vi "Settings Dialog.vi"(8 "error in (no error)":errorcluster, 11 "Settings in":T1={"Logging Configuration"={"Log File Base Path"=path "", "Samples to Save"=0, "Acquisition Sample Rate"=0.0, "SamplesPerChannel"=0, "FFT - Block Size"=0, "FFT - NumberOfAverages"=0, "Trigger - Time"=0, "Trigger - Threshold"=0.0, "Trigger - Channel"=0, "Enable Start Output Trigger"=FALSE, "Enable Time Trigger"=FALSE, "Enable Threshold Trigger"=FALSE, "HasBeenTriggeredAlready"=FALSE, "Always Log"=FALSE, "Enable Filter"=FALSE, "FilesRefs"={"TimeDomainTDMSRef"=refnum, "FrequencyDomainTDMSRef"=refnum, "TimeDomainTXTRef"=refnum, "FrequencyDomainTXTRef "=refnum}, "OutputFileFormat"=enum."TXT", "ActualBlockSize"=0, "Start Time"=timestamp(0 s since 1904-01-01)}, "Hardware Configuration"={"Accel-ai0"=FALSE, "Maximum Input"=0.0, "Minimum Input"=0.0, "HW Sample Rate"=0.0, "SW Sample Rate"=0.0, "Number of Samples"=0, "Accel-ai1"=FALSE, "DAQmx Task"="", "Low Pass Filter"={"Upper Cutoff"=350.0, "Lower Cutoff"=350.0, "Order"=350}}, "Output Hardware Configuration"={"Task ID"=0, "Volume"=0.0, "Sample Rate"=0.0, "Duration"=0, "Data"={"SignalType"=enum."SineWave", "Amplitude"=0.0, "WhiteNoiseSettings"={"Generate New Data"=FALSE, "Save"=FALSE, "Filter"=TRUE, "Gain"=0.0}, "SineWaveSttings"={"Frequency"=0.0}}, "Generated Data"={"t0"=timestamp(0 s since 1904-01-01), "dt"=1.0, "Y"=[]}}} {"Output Hardware Configuration"."task ID out" format="%.0x"; "Hardware Configuration"."Low Pass Filter"."Order" min=0 max=10 step=1}) -> (0 "error out":errorcluster, 1 "Cancelled?":bool=TRUE, 2 "UI Refresh Needed?":bool, 3 "Settings Out":T1={"Logging Configuration"={"Log File Base Path"=path "", "Samples to Save"=0, "Acquisition Sample Rate"=0.0, "SamplesPerChannel"=0, "FFT - Block Size"=0, "FFT - NumberOfAverages"=0, "Trigger - Time"=0, "Trigger - Threshold"=0.0, "Trigger - Channel"=0, "Enable Start Output Trigger"=FALSE, "Enable Time Trigger"=FALSE, "Enable Threshold Trigger"=FALSE, "HasBeenTriggeredAlready"=FALSE, "Always Log"=FALSE, "Enable Filter"=FALSE, "FilesRefs"={"TimeDomainTDMSRef"=refnum, "FrequencyDomainTDMSRef"=refnum, "TimeDomainTXTRef"=refnum, "FrequencyDomainTXTRef "=refnum}, "OutputFileFormat"=enum."TXT", "ActualBlockSize"=0, "Start Time"=timestamp(0 s since 1904-01-01)}, "Hardware Configuration"={"Accel-ai0"=FALSE, "Maximum Input"=0.0, "Minimum Input"=0.0, "HW Sample Rate"=0.0, "SW Sample Rate"=0.0, "Number of Samples"=0, "Accel-ai1"=FALSE, "DAQmx Task"="", "Low Pass Filter"={"Upper Cutoff"=350.0, "Lower Cutoff"=350.0, "Order"=350}}, "Output Hardware Configuration"={"Task ID"=0, "Volume"=0.0, "Sample Rate"=0.0, "Duration"=0, "Data"={"SignalType"=enum."SineWave", "Amplitude"=0.0, "WhiteNoiseSettings"={"Generate New Data"=FALSE, "Save"=FALSE, "Filter"=TRUE, "Gain"=0.0}, "SineWaveSttings"={"Frequency"=0.0}}, "Generated Data"={"t0"=timestamp(0 s since 1904-01-01), "dt"=1.0, "Y"=[]}}} {"Output Hardware Configuration"."task ID out" format="%.0x"; "Hardware Configuration"."Low Pass Filter"."Order" min=0 max=10 step=1})   [LabVIEW 2022 SP3, in "Settings.lvlib"]
doc: "Dialog for selecting user specified settings."
uses:
  Settings.lvlib
  Settings.ctl
  Logging/Logging Configuration.ctl
  support/TDMS-Refs.ctl
  FiniteMeasurement-DAQmx/controls/Hardware Configuration.ctl
  AcquisitionFilter.ctl
  Output/Output Hardware Configuration.ctl
  <vilib>/sound2/lvsound2.llb/Sound Output Task ID.ctl
  Output/Data.ctl
  Output/WhiteNoiseSettings.ctl
  Output/SineWaveSettings.ctl
  <vilib>/Utility/xml.llb/Write to XML File(string).vi
  <resource>/objmgr/daqmx.rc
  Logging/Logging.lvlib
  Acquisition/Acquisition.lvlib
panel:
  out "Frequency Delta(Hz)":dbl
  in  "Logging Configuration.Enable Filter":bool
  in  "Lower Cutoff":dbl
  in  "Order":i32
  in  "Number of FFT Averages":i32=5
  in  "Block Size":u32=100 min=100 max=10240 step=10
  in  "Accelerometer AI-1":bool
  in  "Accelerometer AI-0":bool=TRUE
  in  "Log when triggered":bool
  in  "Trigger Channel":u32
  in  "Timeout (s)":u32=206000 min=1
  in  "Trigger Threshold (V)":dbl=2.0
  in  "Trigger Time (s)":u32=1
  in  "Enable Threshold Trigger (m/s²):":bool
  in  "Enable Time Trigger (s):":bool
  in  "Always Log":bool
  in  "HW Sample Rate":i32=20000 min=1000 max=20000
  in  "SW Sample Rate":dbl=220.0
  in  "Max/Min Input":dbl=5.0
  in  "Log Base Path":path=path "C:/Users/LAV-UFSC-2023/Documents/LAV-TCC/Dados-Experimentos/Dados-Bancada-LABVIEW/teste.txt"
  in  "Cancel Button":bool
  in  "OK Button":bool
  # "Acquisition"
  # "Non visible portion of dialog (needed for connector pane)."
  # "LowPassFilter"
  # "Trigger"
  # "Logging"
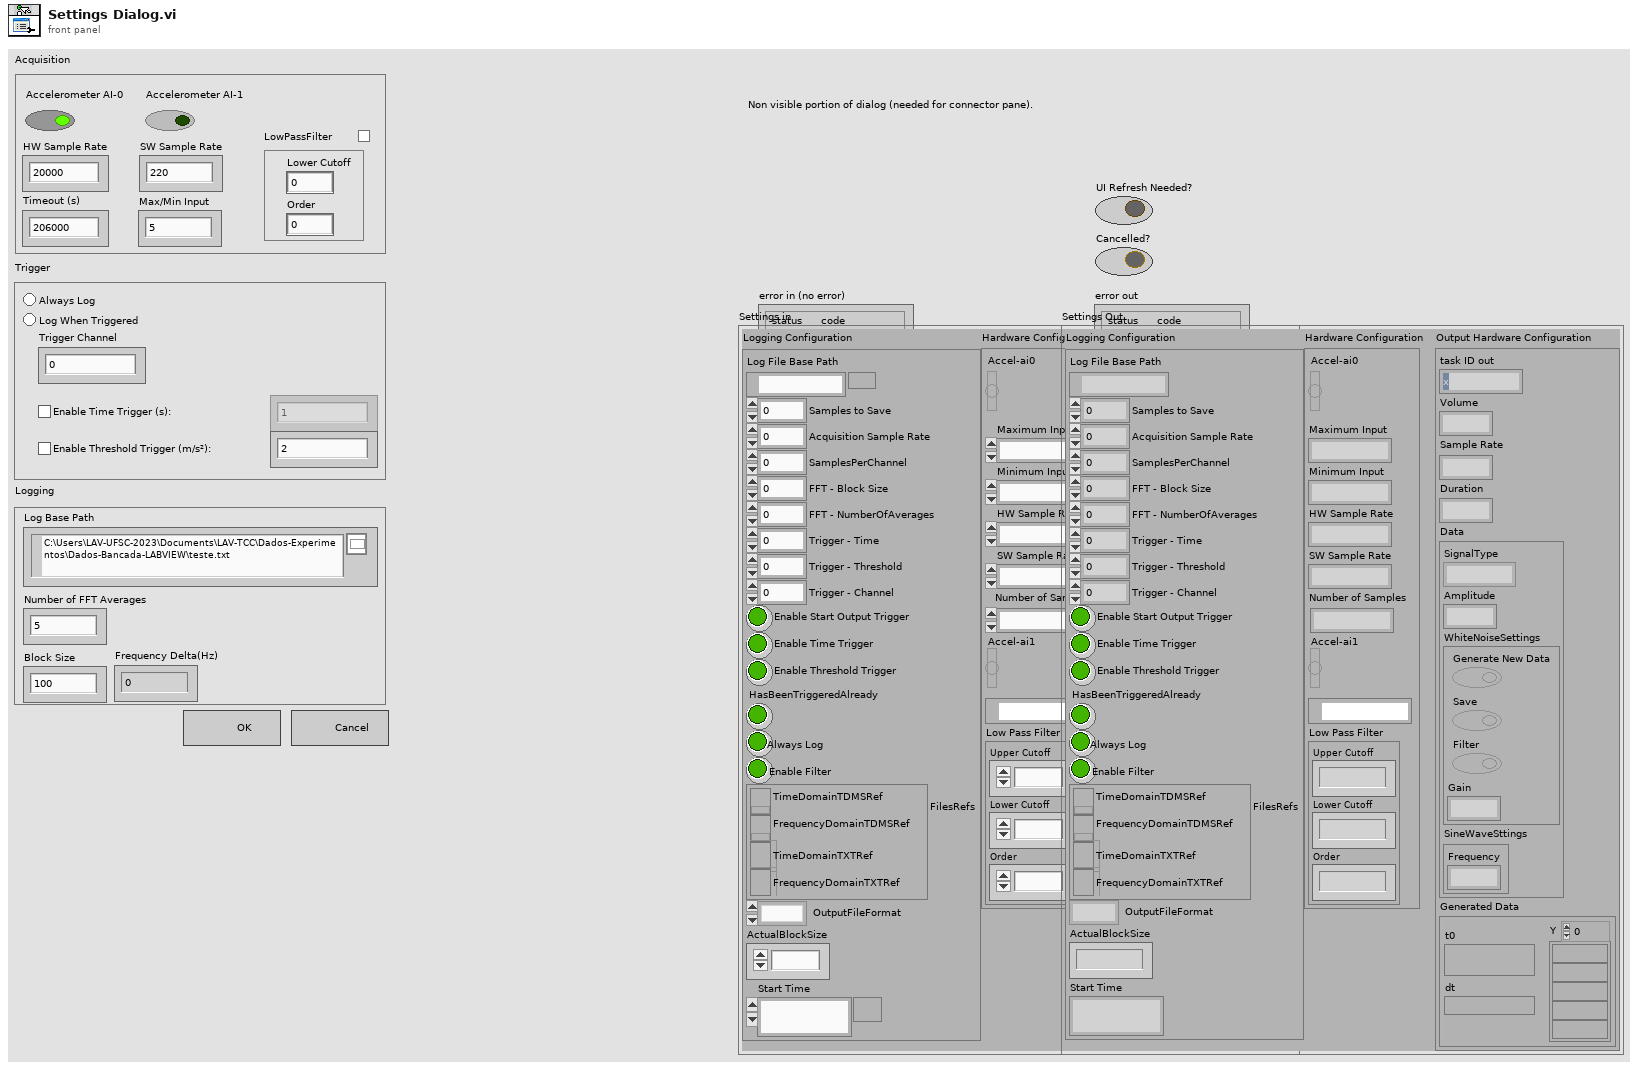
[diagram p1: front panel]
types:
  T1 = typedef "Settings.lvlib/Settings.ctl" = cluster{"Logging Configuration":T2, "Hardware Configuration":T4, "Output Hardware Configuration":T6}
  T2 = typedef "Logging.lvlib/Logging Configuration.ctl" = cluster{"Log File Base Path":path, "Samples to Save":u32, "Acquisition Sample Rate":dbl, "SamplesPerChannel":u32, "FFT - Block Size":u32, "FFT - NumberOfAverages":i32, "Trigger - Time":i32, "Trigger - Threshold":dbl, "Trigger - Channel":i32, "Enable Start Output Trigger":bool, "Enable Time Trigger":bool, "Enable Threshold Trigger":bool, "HasBeenTriggeredAlready":bool, "Always Log":bool, "Enable Filter":bool, "FilesRefs":T3, "OutputFileFormat":enum16{"TXT", "TDMS"}, "ActualBlockSize":i32, "Start Time":timestamp}
  T3 = typedef "TDMS-Refs.ctl" = cluster{"TimeDomainTDMSRef":refnum<k34>, "FrequencyDomainTDMSRef":refnum<k34>, "TimeDomainTXTRef":refnum<file>, "FrequencyDomainTXTRef ":refnum<file>}
  T4 = typedef "Acquisition.lvlib/Hardware Configuration.ctl" = cluster{"Accel-ai0":bool, "Maximum Input":dbl, "Minimum Input":dbl, "HW Sample Rate":dbl, "SW Sample Rate":dbl, "Number of Samples":i32, "Accel-ai1":bool, "DAQmx Task":refnum<k21>, "Low Pass Filter":T5}
  T5 = typedef "Acquisition.lvlib/AcquisitionFilter.ctl" = cluster{"Upper Cutoff":dbl, "Lower Cutoff":dbl, "Order":i32}
  T6 = typedef "Output Hardware Configuration.ctl" = cluster{"Task ID":T7, "Volume":dbl, "Sample Rate":dbl, "Duration":i32, "Data":T8, "Generated Data":waveform(dbl)}
  T7 = typedef "Sound Output Task ID.ctl" = u32
  T8 = typedef "Data.ctl" = cluster{"SignalType":enum16{"WhiteNoise", "SineWave"}, "Amplitude":dbl, "WhiteNoiseSettings":T9, "SineWaveSttings":T10}
  T9 = typedef "WhiteNoiseSettings.ctl" = cluster{"Generate New Data":bool, "Save":bool, "Filter":bool, "Gain":dbl}
  T10 = typedef "SineWaveSettings.ctl" = cluster{"Frequency":dbl}
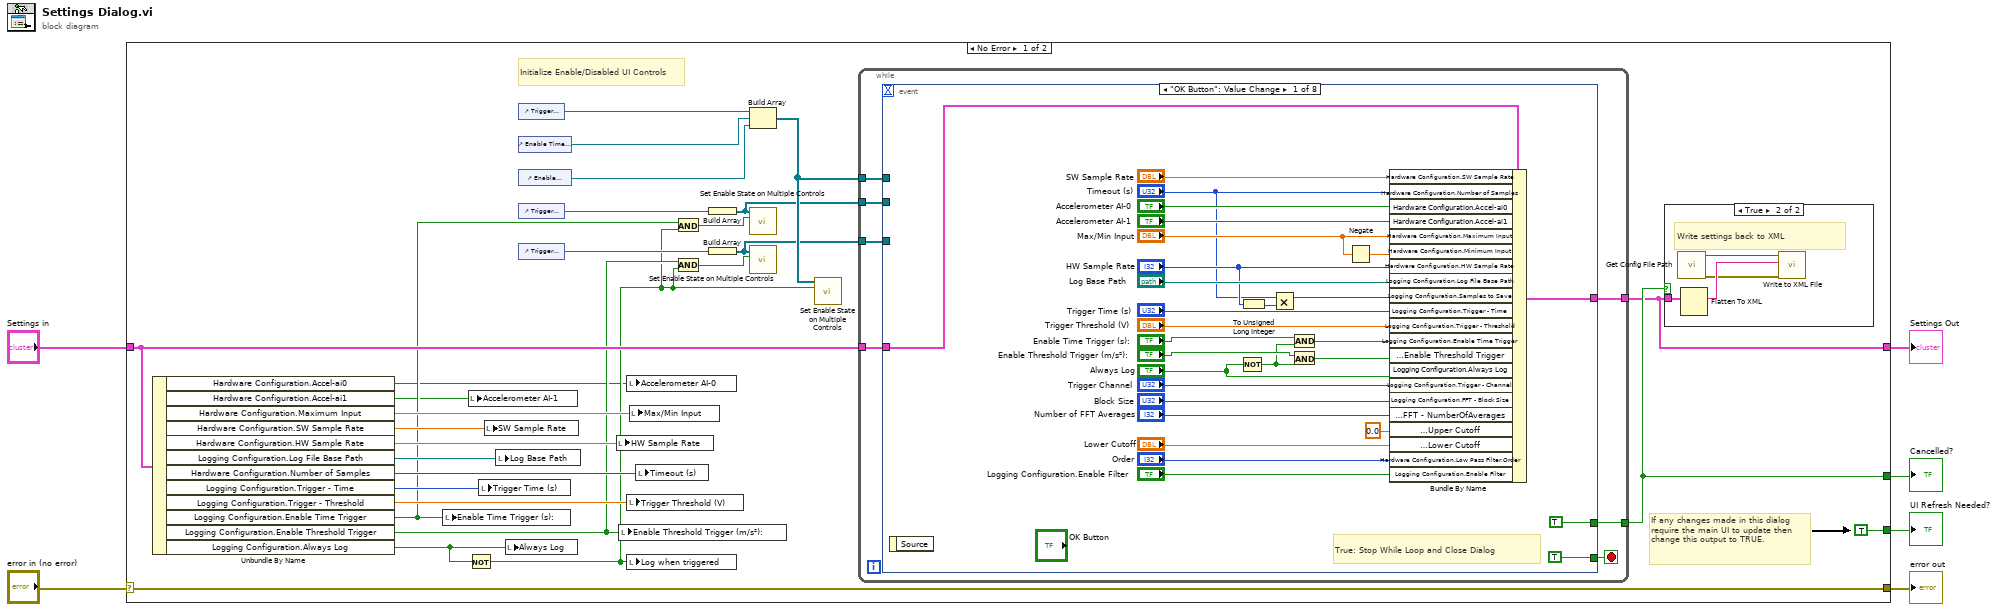
[diagram p0: block diagram]
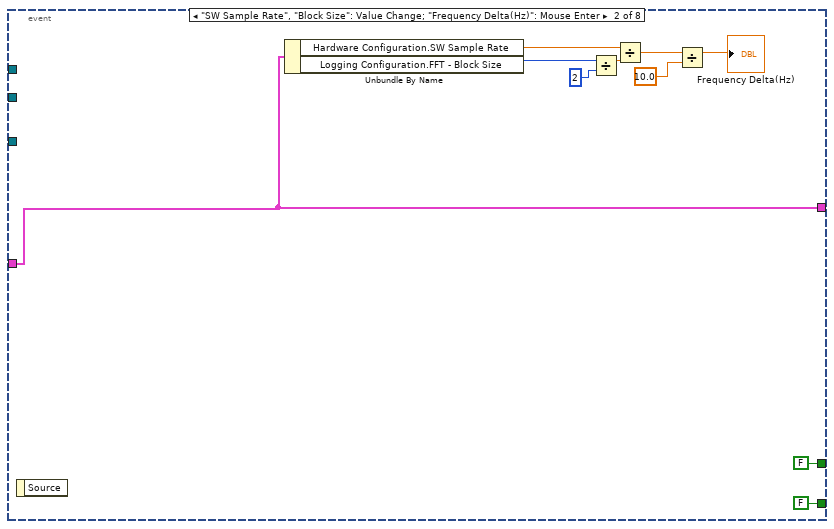
[diagram p2: hidden frame]
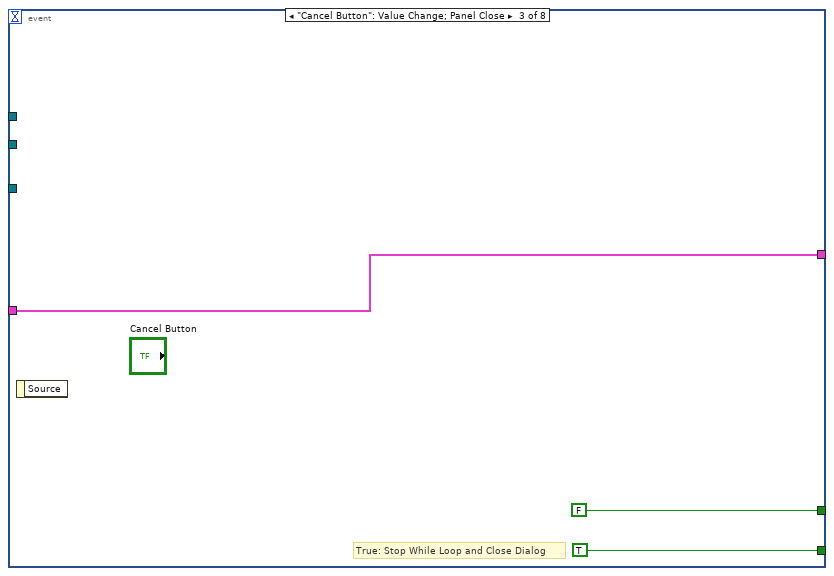
[diagram p3: hidden frame]
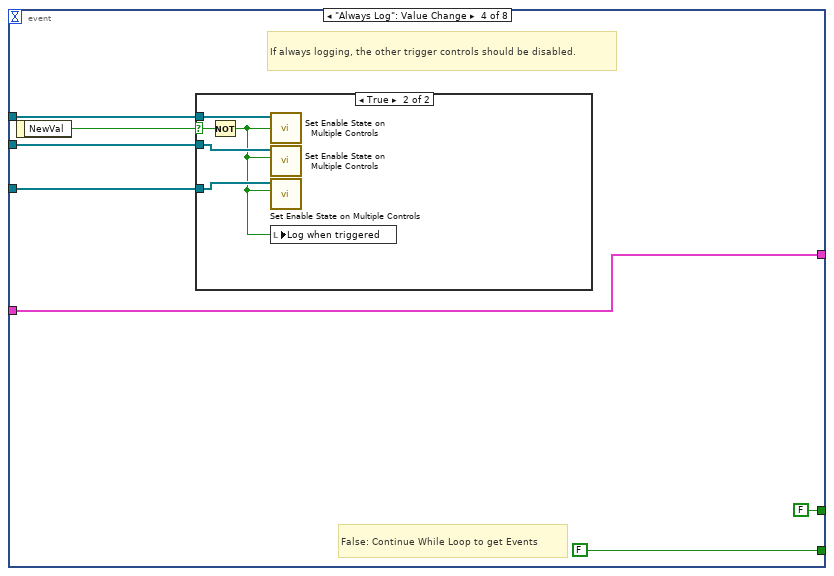
[diagram p4: hidden frame]
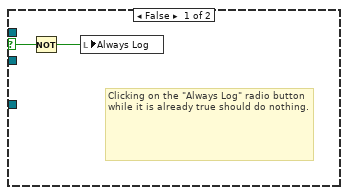
[diagram p5: hidden frame]
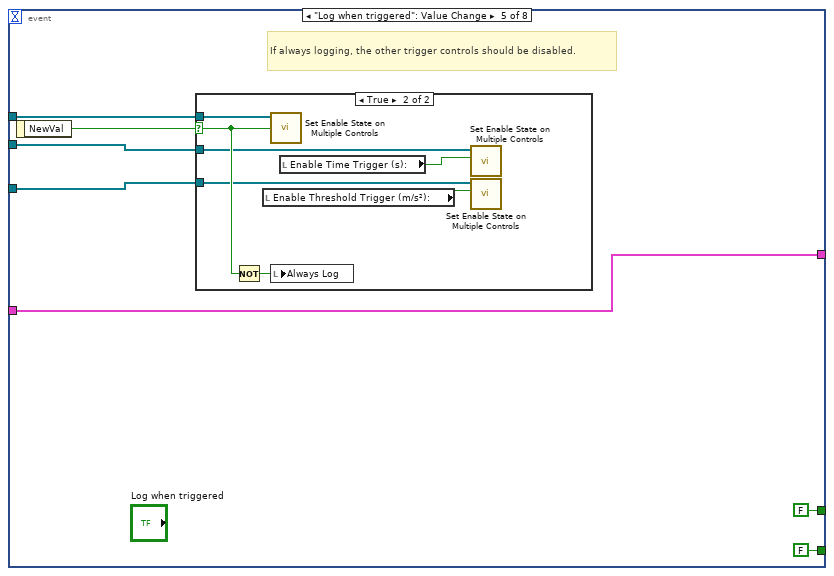
[diagram p6: hidden frame]
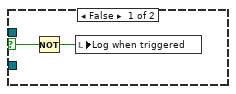
[diagram p7: hidden frame]
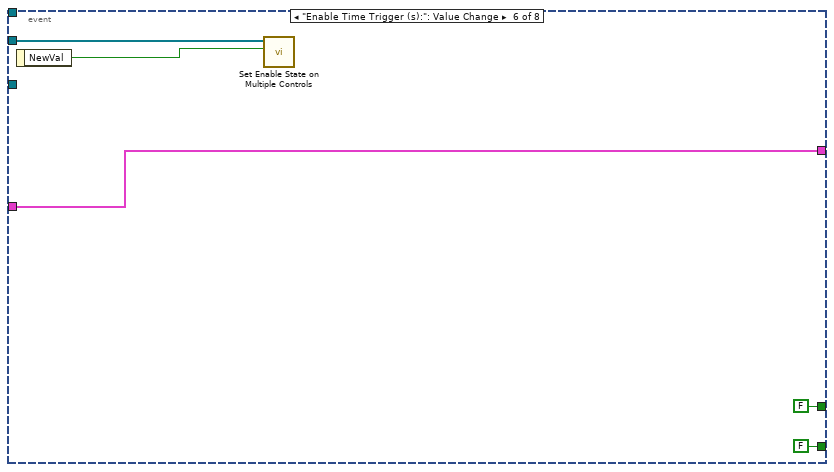
[diagram p8: hidden frame]
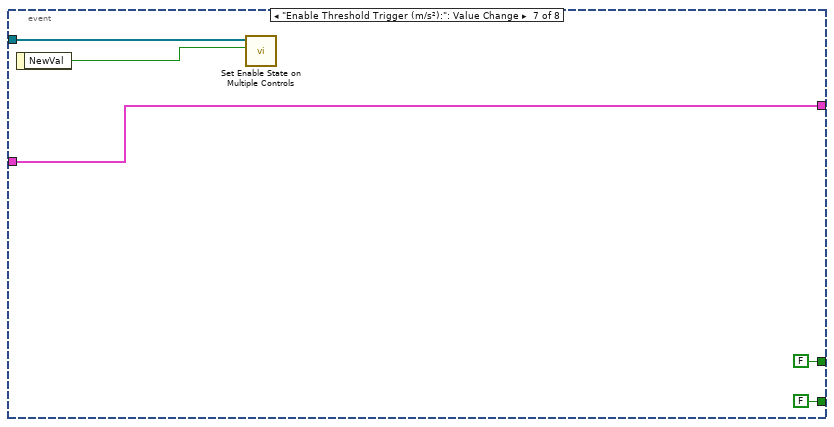
[diagram p9: hidden frame]
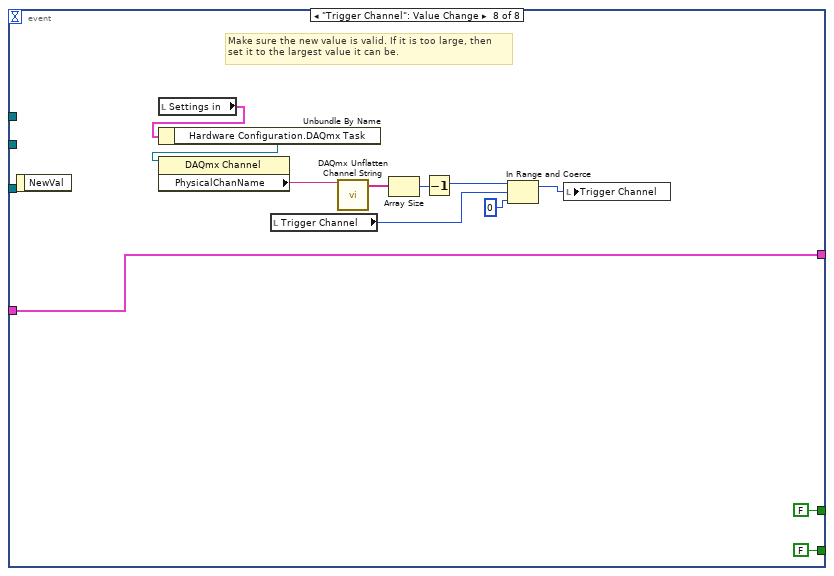
[diagram p10: hidden frame]
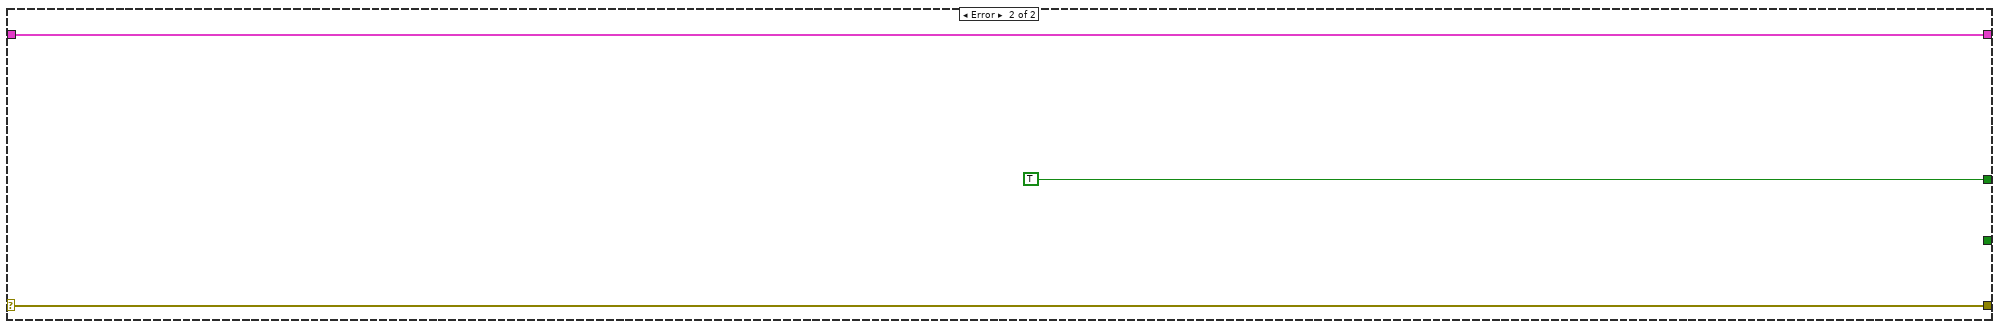
[diagram p12: hidden frame]
diagram:
  n1 = case shown="No Error" "error in (no error)" {
    selector: "error in (no error)" -> [w34 w142]
    tunnel: [w34 w142] -> w6
    tunnel: "Settings in" -> [w21 w141]
    tunnel: [w31 w141] -> w5
    tunnel: [TRUE ("UI Refresh Needed?") _] -> w4
    tunnel: [w32 TRUE ("UI Refresh Needed?")] -> w3
    frame No Error {
      # "Initialize Enable/Disabled UI Controls"
      # "If any changes made in this dialog require the main UI to update then change this output to TRUE."
      n2 = Unbundle By Name(w21) -> ("Hardware Configuration.Accel-ai0"=w7:bool, "Hardware Configuration.Accel-ai1"=w8:bool, "Hardware Configuration.Maximum Input"=w28:dbl, "Hardware Configuration.SW Sample Rate"=w29:dbl, "Hardware Configuration.HW Sample Rate"=w30:dbl, "Logging Configuration.Log File Base Path"=w27:path, "Hardware Configuration.Number of Samples"=w26:i32, "Logging Configuration.Trigger - Time"=w25:i32, "Logging Configuration.Trigger - Threshold"=w24:dbl, "Logging Configuration.Enable Time Trigger"=w13:bool, "Logging Configuration.Enable Threshold Trigger"=w12:bool, "Logging Configuration.Always Log"=w23:bool)
      n3 = local write "Enable Time Trigger (s):"(w13) -> ()
      n4 = Not(x=w23) -> (.not. x?=w9:bool)
      n5 = local write "Accelerometer AI-1"(w8) -> ()
      n6 = local write "Trigger Time (s)"(w25) -> ()
      n7 = local write "SW Sample Rate"(w29) -> ()
      n8 = local write "Log Base Path"(w27) -> ()
      n9 = local write "Always Log"(w23) -> ()
      n10 = control-ref of="Trigger Channel"() -> (w20:refnum<vi>)
      n11 = control-ref of="Enable Time Trigger (s):"() -> (w19:refnum<vi>)
      n12 = control-ref of="Enable Threshold Trigger (m/s²):"() -> (w18:refnum<vi>)
      n13 = control-ref of="Trigger Time (s)"() -> (w17:refnum<vi>)
      n14 = control-ref of="Trigger Threshold (V)"() -> (w16:refnum<vi>)
      n15 = local write "HW Sample Rate"(w30) -> ()
      n16 = local write "Enable Threshold Trigger (m/s²):"(w12) -> ()
      n17 = local write "Accelerometer AI-0"(w7) -> ()
      n18 = local write "Trigger Threshold (V)"(w24) -> ()
      n19 = local write "Log when triggered"(w9) -> ()
      n20 = local write "Max/Min Input"(w28) -> ()
      n21 = local write "Timeout (s)"(w26) -> ()
      n22 = And(x=w13, y=w9) -> (x .and. y?=w15:bool)
      n23 = And(x=w12, y=w9) -> (x .and. y?=w14:bool)
      n24 = Build Array(w17) -> (w11:refnum<vi>[])
      n25 = Build Array(w16) -> (w10:refnum<vi>[])
      n26 = Build Array(w20, w19, w18) -> (w22:refnum<vi>[])
      n27 = call "Set Enable State on Multiple Controls.vi"("Enable?"=w15, "Controls"=w11) -> ()  [unwired: 10 in]
      n28 = call "Set Enable State on Multiple Controls.vi"("Enable?"=w14, "Controls"=w10) -> ()  [unwired: 10 in]
      n29 = call "Set Enable State on Multiple Controls.vi"("Enable?"=w9, "Controls"=w22) -> ()  [unwired: 10 in]
      n30 = while {
        tunnel: [w41] -> w32
        tunnel: [w40] -> w31
        tunnel: w21 -> [w39]
        tunnel: w22 -> [w37]
        tunnel: w11 -> [w36]
        tunnel: w10 -> [w35]
        stop <- w38 stop-if-true
        n31 = event shown="[0] \"OK Button\": Value Change" {
          selector: _ -> [_ _ _ _ _ _ _ _]
          dyn-events: _ -> [_ _ _ _ _ _ _ _]
          timeout: _ -> [_ _ _ _ _ _ _ _]
          tunnel: [w68 w80 w83 w90 w104 w118 w123 w135] -> w40
          tunnel: w39 -> [w67 w80 w83 w90 w104 w118 w123 w135]
          tunnel: [TRUE ("UI Refresh Needed?") FALSE ("UI Refresh Needed?") FALSE ("UI Refresh Needed?") FALSE ("UI Refresh Needed?") FALSE ("UI Refresh Needed?") FALSE ("UI Refresh Needed?") FALSE ("UI Refresh Needed?") FALSE ("UI Refresh Needed?")] -> w41
          tunnel: [TRUE FALSE TRUE FALSE FALSE FALSE FALSE FALSE] -> w38
          tunnel: w37 -> [_ _ _ w88 w103 _ _ _]
          tunnel: w36 -> [_ _ _ w86 w101 w117 _ _]
          tunnel: w35 -> [_ _ _ w85 w100 _ w122 _]
          event "OK Button": Value Change {
            # "True: Stop While Loop and Close Dialog"
            n32 = event-data() -> ()  [unwired: 1 in, 1 out]
            n33 = Not(x="Always Log") -> (.not. x?=w57:bool)
            n34 = To Unsigned Long Integer(number="HW Sample Rate") -> (unsigned 32bit integer=w45:u32)
            n35 = Multiply(x="Timeout (s)", y=w45) -> (x*y=w42:u32)
            n36 = And(x="Enable Time Trigger (s):", y=w57) -> (x .and. y?=w58:bool)
            n37 = And(x="Enable Threshold Trigger (m/s²):", y=w57) -> (x .and. y?=w60:bool)
            n38 = Negate(x="Max/Min Input") -> (-x=w48:dbl)
            n39 = Bundle By Name(cluster=w67, "Hardware Configuration.SW Sample Rate"="SW Sample Rate", "Hardware Configuration.Number of Samples"="Timeout (s)", "Hardware Configuration.Accel-ai0"="Accelerometer AI-0", "Hardware Configuration.Accel-ai1"="Accelerometer AI-1", "Hardware Configuration.Maximum Input"="Max/Min Input", "Hardware Configuration.Minimum Input"=w48, "Hardware Configuration.HW Sample Rate"="HW Sample Rate", "Logging Configuration.Log File Base Path"="Log Base Path", "Logging Configuration.Samples to Save"=w42, "Logging Configuration.Trigger - Time"="Trigger Time (s)", "Logging Configuration.Trigger - Threshold"="Trigger Threshold (V)", "Logging Configuration.Enable Time Trigger"=w58, "Logging Configuration.Enable Threshold Trigger"=w60, "Logging Configuration.Always Log"="Always Log", "Logging Configuration.Trigger - Channel"="Trigger Channel", "Logging Configuration.FFT - Block Size"="Block Size", "Logging Configuration.FFT - NumberOfAverages"="Number of FFT Averages", "Hardware Configuration.Low Pass Filter.Upper Cutoff"=0.0, "Hardware Configuration.Low Pass Filter.Lower Cutoff"="Lower Cutoff", "Hardware Configuration.Low Pass Filter.Order"="Order", "Logging Configuration.Enable Filter"="Logging Configuration.Enable Filter") -> (w68:T1)
          }
          event "SW Sample Rate", "Block Size": Value Change; "Frequency Delta(Hz)": Mouse Enter {
            n40 = event-data() -> ()  [unwired: 1 in, 1 out]
            n41 = Unbundle By Name(w80) -> ("Hardware Configuration.SW Sample Rate"=w79:dbl, "Logging Configuration.FFT - Block Size"=w78:u32)
            n42 = Divide(x=w78, y=u32 2) -> (x/y=w74:dbl)
            n43 = Divide(x=w79, y=w74) -> (x/y=w77:dbl)
            n44 = Divide(x=w77, y=10.0) -> (x/y=→"Frequency Delta(Hz)":dbl)
          }
          event "Cancel Button": Value Change; Panel Close {
            # "True: Stop While Loop and Close Dialog"
            n45 = event-data() -> ()  [unwired: 1 in, 1 out]
          }
          event "Always Log": Value Change {
            # "False: Continue While Loop to get Events"
            # "If always logging, the other trigger controls should be disabled."
            n46 = event-data() -> ("NewVal"=w87:bool)  [unwired: 1 in]
            n47 = case shown="True" w87 {
              selector: w87 -> [w92 w97]
              tunnel: w88 -> [_ w96]
              tunnel: w86 -> [_ w95]
              tunnel: w85 -> [_ w94]
              frame False {
                # "Clicking on the \"Always Log\" radio button while it is already true should do nothing."
                n48 = Not(x=w92) -> (.not. x?=w91:bool)
                n49 = local write "Always Log"(w91) -> ()
              }
              frame True {
                n50 = Not(x=w97) -> (.not. x?=w93:bool)
                n51 = call "Set Enable State on Multiple Controls.vi"("Enable?"=w93, "Controls"=w96) -> ()  [unwired: 10 in]
                n52 = call "Set Enable State on Multiple Controls.vi"("Enable?"=w93, "Controls"=w95) -> ()  [unwired: 10 in]
                n53 = call "Set Enable State on Multiple Controls.vi"("Enable?"=w93, "Controls"=w94) -> ()  [unwired: 10 in]
                n54 = local write "Log when triggered"(w93) -> ()
              }
            }
          }
          event "Log when triggered": Value Change {
            # "If always logging, the other trigger controls should be disabled."
            n55 = event-data() -> ("NewVal"=w102:bool)  [unwired: 1 in]
            n56 = case shown="True" w102 {
              selector: w102 -> [w106 w112]
              tunnel: w103 -> [_ w113]
              tunnel: w101 -> [_ w110]
              tunnel: w100 -> [_ w109]
              frame False {
                n57 = Not(x=w106) -> (.not. x?=w105:bool)
                n58 = local write "Log when triggered"(w105) -> ()
              }
              frame True {
                n59 = Not(x=w112) -> (.not. x?=w111:bool)
                n60 = local read "Enable Threshold Trigger (m/s²):"() -> (w108:bool)
                n61 = call "Set Enable State on Multiple Controls.vi"("Enable?"=w112, "Controls"=w113) -> ()  [unwired: 10 in]
                n62 = local write "Always Log"(w111) -> ()
                n63 = local read "Enable Time Trigger (s):"() -> (w107:bool)
                n64 = call "Set Enable State on Multiple Controls.vi"("Enable?"=w107, "Controls"=w110) -> ()  [unwired: 10 in]
                n65 = call "Set Enable State on Multiple Controls.vi"("Enable?"=w108, "Controls"=w109) -> ()  [unwired: 10 in]
              }
            }
          }
          event "Enable Time Trigger (s):": Value Change {
            n66 = event-data() -> ("NewVal"=w116:bool)  [unwired: 1 in]
            n67 = call "Set Enable State on Multiple Controls.vi"("Enable?"=w116, "Controls"=w117) -> ()  [unwired: 10 in]
          }
          event "Enable Threshold Trigger (m/s²):": Value Change {
            n68 = event-data() -> ("NewVal"=w121:bool)  [unwired: 1 in]
            n69 = call "Set Enable State on Multiple Controls.vi"("Enable?"=w121, "Controls"=w122) -> ()  [unwired: 10 in]
          }
          event "Trigger Channel": Value Change {
            # "Make sure the new value is valid. If it is too large, then\nset it to the largest value it can be."
            n70 = event-data() -> ()  [unwired: 1 in, 1 out]
            n71 = local read "Settings in"() -> (w128:T1)
            n72 = Unbundle By Name(w128) -> ("Hardware Configuration.DAQmx Task"=w127:refnum<k21>)
            n73 = property class="DAQmx Channel"(reference=w127) -> ("PhysicalChanName"=w126:tag)  [unwired: 1 in, 2 out]
            n74 = local read "Trigger Channel"() -> (w129:u32)
            n75 = call <vilib>:"DAQmx Unflatten Channel String.vi"("names in"=w126) -> ("names out"=w134:string[])  [unwired: 13 in, 1 out]
            n76 = Array Size(array=w134) -> (size(s)=w133:i32)
            n77 = Decrement(x=w133) -> (x-1=w132:i32)
            n78 = In Range and Coerce(upper limit=w132, x=w129, lower limit=u32 0) -> (coerced(x)=w130:u32)  [unwired: 1 out]
            n79 = local write "Trigger Channel"(w130) -> ()
          }
        }
      }
      n80 = case shown="True" w32 {
        tunnel: w31 -> [_ w138]
        frame False {
        }
        frame True {
          # "Write settings back to XML"
          n81 = call "Get Config File Path.vi"() -> ("error out"=w136:errorcluster, "XML File Path"=w139:path)  [unwired: 10 in]
          n82 = Flatten To XML(6:w138) -> (2:w137:string)
          n83 = call-poly <vilib>:"Write to XML File.vi"("error in (no error)"=w136, "XML Input"=w137, "XML File Path"=w139) -> ()  [unwired: 6 in, 3 out]
        }
      }
    }
    frame Error {
    }
  }
  "UI Refresh Needed?" <- w4
  "error out" <- w6
  "Cancelled?" <- w3
  "Settings Out" <- w5
